vi "zad1.vi"() -> ()   [LabVIEW 2018]
uses:
  <vilib>/Utility/miscctls.llb/LV3DPointTypeDef.ctl
  <vilib>/picture/3D Picture Control/Object/Create Object (drawable).vi
  <vilib>/picture/3D Picture Control/Object/Add Object (reference).vi
  <vilib>/picture/3D Picture Control/NI_3D Picture Control.lvlib
panel:
  in  "Translation":T1
  out "3D Picture":refnum<vi>(3d-picture)
  in  "stop":bool
  in  "Angle 2":sgl
  in  "Axis 2":T1
  in  "Angle":sgl
  in  "Axis":T1
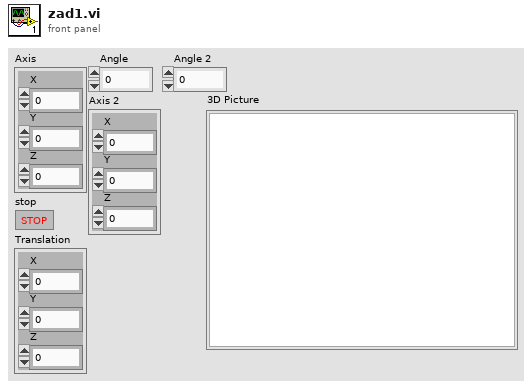
[diagram p1: front panel]
types:
  T1 = typedef "LV3DPointTypeDef.ctl" = cluster{"X":sgl, "Y":sgl, "Z":sgl}
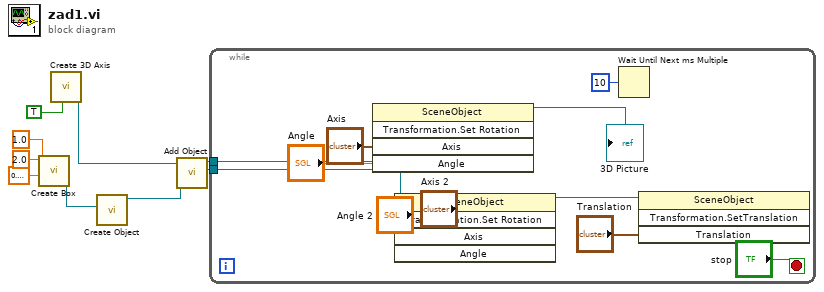
[diagram p0: block diagram]
diagram:
  n1 = call <vilib>:"Create Box.vi"("Length Z"=sgl 0.1, "Length Y"=sgl 1.0, "Length X"=sgl 2.0) -> ("New Box Refnum"=w2:refnum<vi>)  [unwired: 7 in, 1 out]
  n2 = call <vilib>:"Create 3D Axis.vi"("Axis label?"=TRUE) -> ("New Object Refnum"=w9:refnum<vi>)  [unwired: 9 in, 1 out]
  n3 = call-poly <vilib>:"Create Object.vi"("Geometry"=w2) -> ("Scene:New Object"=w8:refnum<vi>)  [unwired: 9 in, 1 out]
  n4 = call-poly <vilib>:"Add Object.vi"("New Object In"=w8, "Scene Object In"=w9) -> ("New Object Out"=w1:refnum<vi>, "Scene Object Out"=w7:refnum<vi>)  [unwired: 7 in, 1 out]
  n5 = while {
    tunnel: w7 -> [w19]
    tunnel: w1 -> [w20]
    stop <- "stop" stop-if-true
    n6 = invoke class="SceneObject" method="Transformation.Set Rotation"(reference=w19, "Axis"="Axis", "Angle"="Angle") -> (reference out=→"3D Picture":refnum<vi>)  [unwired: 2 in, 4 out]
    n7 = invoke class="SceneObject" method="Transformation.Set Rotation"(reference=w20, "Axis"="Axis 2", "Angle"="Angle 2") -> (reference out=w12:refnum<vi>)  [unwired: 2 in, 4 out]
    n8 = Wait Until Next ms Multiple(millisecond multiple=u32 10) -> ()  [unwired: 1 out]
    n9 = invoke class="SceneObject" method="Transformation.SetTranslation"(reference=w12, "Translation"="Translation") -> ()  [unwired: 2 in, 4 out]
  }
